vi "button no button.vi"() -> ()   [LabVIEW 2021]
uses:
  <vilib>/myRIO/Instrument Drivers/Onboard IO/PWM/typedefs/PWM Reference.ctl
  <vilib>/myRIO/Common/Instrument Driver Framework/Utilities/typedefs/myRIO Generic Hardware Reference.ctl
  <vilib>/myRIO/Common/Instrument Driver Framework/Utilities/typedefs/Hardware Version Enum.ctl
  <vilib>/myRIO/Common/Instrument Driver Framework/Utilities/typedefs/myRIO v1.0 Reference.ctl
  <vilib>/myRIO/Common/Instrument Driver Framework/Utilities/typedefs/Generic FPGA Reference.ctl
  <vilib>/myRIO/Common/Instrument Driver Framework/myRIO v1.0/PWM/typedefs/PWM Channels Enum.ctl
  <vilib>/myRIO/Instrument Drivers/Onboard IO/PWM/typedefs/PWM Configuration.ctl
  <vilib>/userDefined/High Color/nirio_resource_hc.ctl
  <vilib>/myRIO/Instrument Drivers/Onboard IO/DIO/typedefs/DIO Reference.ctl
  <vilib>/myRIO/Common/Instrument Driver Framework/myRIO v1.0/DIO/typedefs/DIO Channels List.ctl
  <vilib>/myRIO/Common/Instrument Driver Framework/myRIO v1.0/DIO/typedefs/DIO Channels Enum.ctl
  <vilib>/myRIO/Common/Instrument Driver Framework/myRIO v1.0/PWM/vis/myRIO v1.1 Open PWM.vi
  <vilib>/myRIO/Common/Instrument Driver Framework/myRIO v1.0/DIO/vis/myRIO v1.1 Open DIO.vi
  <vilib>/myRIO/Common/Instrument Driver Framework/Utilities/vis/Validate Channels.vi
  <vilib>/myRIO/Common/Instrument Driver Framework/myRIO v1.0/PWM/vis/myRIO v1.0 Reserve PWM.vi
  <vilib>/myRIO/Instrument Drivers/Onboard IO/PWM/vis/Set Duty Cycle and Frequency.vi
  <vilib>/myRIO/Common/Instrument Driver Framework/myRIO v1.0/DIO/vis/myRIO v1.0 Reserve DIO.vi
  <vilib>/myRIO/Common/Instrument Driver Framework/myRIO v1.0/PWM/vis/myRIO v1.0 Close PWM.vi
  <vilib>/myRIO/Common/Instrument Driver Framework/myRIO v1.0/DIO/vis/myRIO v1.0 Close DIO.vi
  <vilib>/myRIO/Common/Instrument Driver Framework/myRIO v1.0/PWM/vis/myRIO v1.0 Build MUX Configuration PWM.vi
  <vilib>/myRIO/Common/Instrument Driver Framework/myRIO v1.0/Resource Manager/vis/myRIO v1.0 Reserve Channel List.vi
  <vilib>/myRIO/Common/Instrument Driver Framework/myRIO v1.0/DIO/vis/myRIO v1.0 Build MUX Configuration DIO.vi
  <vilib>/myRIO/Common/Instrument Driver Framework/myRIO v1.0/PWM/vis/myRIO v1.0 Unreserve PWM.vi
  <vilib>/myRIO/Common/Instrument Driver Framework/myRIO v1.0/DIO/vis/myRIO v1.0 Unreserve DIO.vi
  <vilib>/myRIO/Common/Instrument Driver Framework/myRIO v1.0/Resource Manager/vis/myRIO v1.0 Create Configuration List.vi
  <vilib>/myRIO/Common/Instrument Driver Framework/myRIO v1.0/Resource Manager/vis/myRIO v1.0 Reserve Channel.vi
  <vilib>/myRIO/Common/Instrument Driver Framework/myRIO v1.0/Resource Manager/vis/myRIO v1.0 Unreserve Channel.vi
  <vilib>/myRIO/Common/Instrument Driver Framework/myRIO v1.0/Resource Manager/vis/myRIO v1.0 Unreserve Channel List.vi
  <vilib>/myRIO/Common/Instrument Driver Framework/myRIO v1.0/Resource Manager/vis/myRIO v1.0 Build Mutex Name.vi
  <vilib>/Utility/VariantDataType/GetNumericInfo.vi
  <vilib>/Utility/error.llb/Error Cluster From Error Code.vi
  <vilib>/myRIO/Common/Instrument Driver Framework/myRIO v1.0/myRIO v1.1 Open.vi
  <vilib>/myRIO/Common/Instrument Driver Framework/Utilities/vis/IO Manager.vi
  <vilib>/myRIO/Common/Instrument Driver Framework/Utilities/vis/Configuration Manager.vi
  <vilib>/myRIO/Common/Instrument Driver Framework/myRIO v1.0/Resource Manager/vis/myRIO v1.0 Configure IO.vi
  <vilib>/myRIO/Common/Instrument Driver Framework/myRIO v1.0/myRIO v1.0 Close.vi
  <vilib>/myRIO/Common/Instrument Driver Framework/myRIO v1.0/PWM/vis/myRIO v1.0 Write PWM.vi
  <vilib>/myRIO/Common/Instrument Driver Framework/myRIO v1.0/DIO/vis/myRIO v1.0 Read DIO.vi
  <vilib>/myRIO/Common/Instrument Driver Framework/myRIO v1.0/PWM/vis/myRIO v1.0 Shutdown PWM.vi
  <vilib>/myRIO/Common/Instrument Driver Framework/myRIO v1.0/DIO/vis/myRIO v1.0 Shutdown DIO.vi
  <vilib>/myRIO/Instrument Drivers/Onboard IO/DIO/vis/myRIO DIO Open.xnode
  <vilib>/myRIO/Instrument Drivers/Onboard IO/PWM/vis/myRIO PWM Open.xnode
  <vilib>/myRIO/Instrument Drivers/Onboard IO/DIO/DIO.lvlib
  <vilib>/myRIO/Instrument Drivers/Onboard IO/PWM/PWM.lvlib
panel:
  in  "error in (no error)":errorcluster
  out "and result":bool
  out "x .and. y?":bool
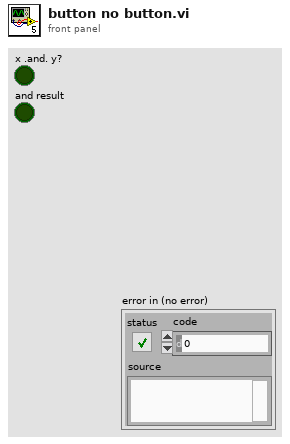
[diagram p1: front panel]
types:
  T1 = typedef "PWM.lvlib/PWM Reference.ctl" = cluster{"myRIO Reference":T2, "PWM Channels Enum":T6, "PWM Configuration":T7}
  T2 = typedef "myRIO Generic Hardware Reference.ctl" = cluster{"myRIO Model":T3, "myRIO Hardware Reference":T4}
  T3 = typedef "Hardware Version Enum.ctl" = enum16{"Unknown", "myRIO-1900", "myRIO-1950", "roboRIO", "NI ELVIS RIO CM", "ELVIS III"}
  T4 = typedef "myRIO v1.0 Reference.ctl" = cluster{"Generic FPGA Reference":T5, "Allow multiple opens":bool}
  T5 = typedef "Generic FPGA Reference.ctl" = refnum<k20>
  T6 = typedef "PWM Channels Enum.ctl" = enum16{"Not Connected", "C/PWM0", "C/PWM1", "A/PWM0", "A/PWM1", "A/PWM2", "A/PWM3", "A/PWM4", "A/PWM5", "A/PWM6", "A/PWM7", "A/PWM8", "A/PWM9", "A/PWM10", "A/PWM11", "A/PWM12", "A/PWM13", "A/PWM14", "A/PWM15", "A/PWM16", "A/PWM17", "A/PWM18", "A/PWM19", "B/PWM0", "B/PWM1", "B/PWM2", "B/PWM3", "B/PWM4", "B/PWM5", "B/PWM6", "B/PWM7", "B/PWM8", "B/PWM9", "B/PWM10", "B/PWM11", "B/PWM12", "B/PWM13", "B/PWM14", "B/PWM15", "B/PWM16", "B/PWM17", "B/PWM18", "B/PWM19", "PWM/PWM0", "PWM/PWM1", "PWM/PWM2", "PWM/PWM3", "PWM/PWM4", "PWM/PWM5", "PWM/PWM6", "PWM/PWM7", "PWM/PWM8", "PWM/PWM9"}
  T7 = typedef "PWM.lvlib/PWM Configuration.ctl" = cluster{"Frequency":dbl, "Duty Cycle":dbl}
  T8 = typedef "DIO.lvlib/DIO Reference.ctl" = cluster{"myRIO Reference":T2, "DIO Channels List":T9}
  T9 = typedef "DIO Channels List.ctl" = T10[]
  T10 = typedef "DIO Channels Enum.ctl" = enum16{"Not Connected", "C/DIO0", "C/DIO1", "C/DIO2", "C/DIO3", "C/DIO4", "C/DIO5", "C/DIO6", "C/DIO7", "A/DIO0", "A/DIO1", "A/DIO2", "A/DIO3", "A/DIO4", "A/DIO5", "A/DIO6", "A/DIO7", "A/DIO8", "A/DIO9", "A/DIO10", "A/DIO11", "A/DIO12", "A/DIO13", "A/DIO14", "A/DIO15", "A/DIO16", "A/DIO17", "A/DIO18", "A/DIO19", "B/DIO0", "B/DIO1", "B/DIO2", "B/DIO3", "B/DIO4", "B/DIO5", "B/DIO6", "B/DIO7", "B/DIO8", "B/DIO9", "B/DIO10", "B/DIO11", "B/DIO12", "B/DIO13", "B/DIO14", "B/DIO15", "B/DIO16", "B/DIO17", "B/DIO18", "B/DIO19", "LED0", "LED1", "LED2", "LED3", "Button0", "DIO/DIO0", "DIO/DIO1", "DIO/DIO2", "DIO/DIO3", "DIO/DIO4", "DIO/DIO5", "DIO/DIO6", "DIO/DIO7", "DIO/DIO8", "DIO/DIO9", "SPI/CS0", "SPI/CS1", "SPI/CS2", "SPI/CS3", "LED RADIO (Green)", "LED RADIO (Red)", "LED COMM (Green)", "LED COMM (Red)", "LED MODE (Green)", "LED MODE (Red)"}
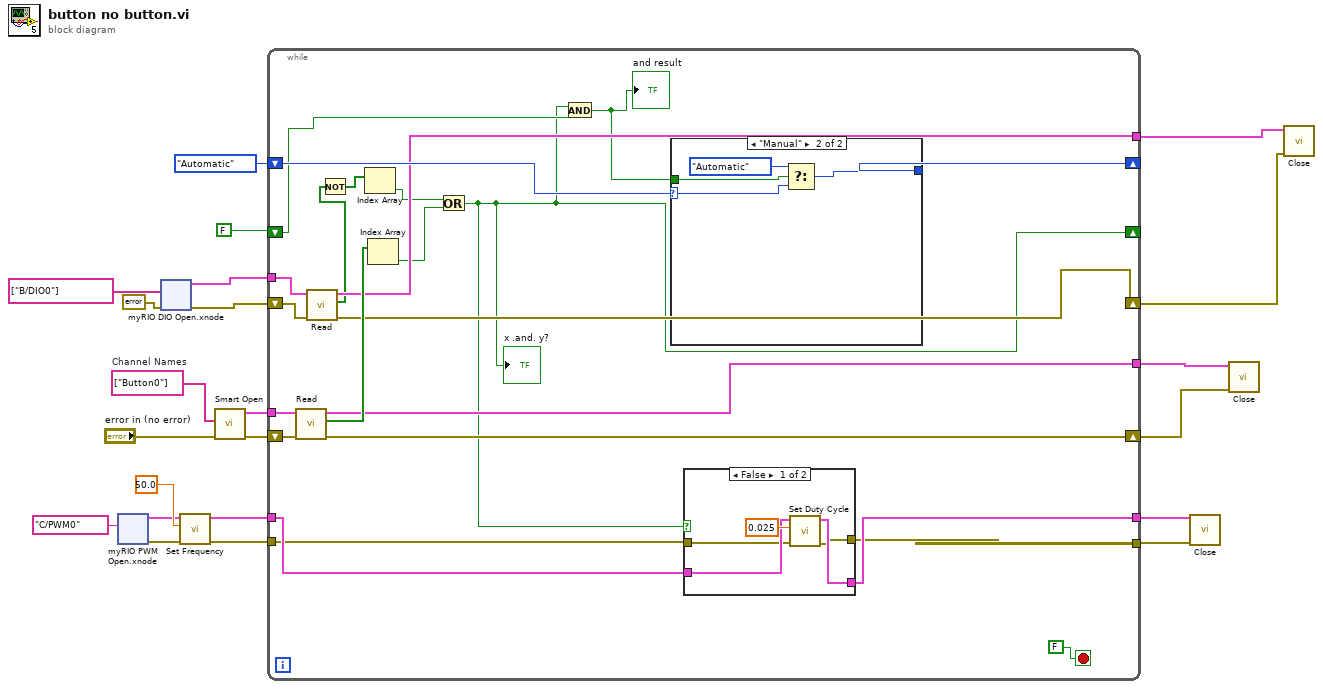
[diagram p0: block diagram]
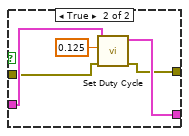
[diagram p2: hidden frame]
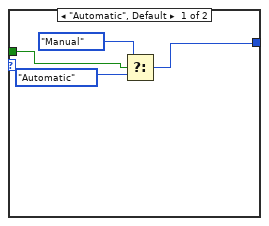
[diagram p3: hidden frame]
diagram:
  w19 = tag[] ["Button0"]  # Channel Names
  n1 = xnode "myRIO PWM Open.xnode"("Channel Name"=tag "C/PWM0") -> ("error out"=w6:errorcluster, "PWM Ref Out"=w7:T1)  [unwired: 2 in]
  n2 = xnode ("myRIO DIO Open.xnode")("error in (no error)"=errorcluster {"status"=FALSE, "code"=0, "source"=""}, "Channel Names"=tag[] ["B/DIO0"]) -> ("error out"=w20:errorcluster, "DIO Ref Out"=w10:T8)  [unwired: 1 in]
  n3 = call <vilib>:"Set Frequency.vi"("error in (no error)"=w6, "Frequency [Hz]"=50.0, "PWM Ref In"=w7) -> ("error out"=w4:errorcluster, "PWM Ref Out"=w5:T1)  [unwired: 6 in]
  n4 = call <vilib>:"Smart Open.vi"("error in (no error)"="error in (no error)", "Channel Names"=w19) -> ("error out"=w22:errorcluster, "DIO Ref Out"=w11:T8)  [unwired: 8 in]
  n5 = while {
    shift-right: [w41] -> w14
    shift-left: w22 -> [w42]
    shift-right: [w34] -> w13
    shift-left: w20 -> [w45]
    tunnel: w10 -> [w44]
    tunnel: w11 -> [w43]
    shift-right: [w38] -> _
    shift-left: enum16{"Automatic", "Manual"}."Automatic" -> [w40]
    tunnel: [w36] -> w16
    tunnel: [w35] -> w15
    tunnel: w5 -> [w24]
    tunnel: w4 -> [w23]
    tunnel: [w26] -> w3
    tunnel: [w25] -> w2
    shift-right: [w27] -> _
    shift-left: FALSE -> [w28]
    stop <- FALSE stop-if-true
    n6 = call <vilib>:"Read.vi"("error in (no error)"=w42, "DIO Ref In"=w43) -> ("error out"=w41:errorcluster, "Values"=w39:bool[], "DIO Ref Out"=w35:T8)  [unwired: 7 in]
    n7 = call <vilib>:"Read.vi"("error in (no error)"=w45, "DIO Ref In"=w44) -> ("error out"=w34:errorcluster, "Values"=w32:bool[], "DIO Ref Out"=w36:T8)  [unwired: 7 in]
    n8 = Not(x=w32) -> (.not. x?=w33:bool[])
    n9 = Index Array "Index Array"(array=w33) -> (element=w29:bool)  [unwired: 1 in]
    n10 = Index Array(array=w39) -> (element=w30:bool)  [unwired: 1 in]
    n11 = Or(x=w29, y=w30) -> (x .or. y?=w27:bool)
    "x .and. y?" <- w27
    n12 = And(x=w27, y=w28) -> (x .and. y?=w31:bool)
    "and result" <- w31
    n13 = case shown="\"Manual\"" w40 {
      selector: w40 -> [_ w61]
      tunnel: [w59 w62] -> w38
      tunnel: w31 -> [w56 w60]
      frame "Automatic", Default {
        n14 = Select(t=enum16{"Automatic", "Manual"}."Manual", s=w56, f=enum16{"Automatic", "Manual"}."Automatic") -> (s? t:f=w59:enum16{"Automatic", "Manual"})
      }
      frame "Manual" {
        n15 = Select(t=enum16{"Automatic", "Manual"}."Automatic", s=w60, f=w61) -> (s? t:f=w62:enum16{"Automatic", "Manual"})
      }
    }
    n16 = case shown="False" w27 {
      tunnel: w24 -> [w49 w54]
      tunnel: w23 -> [w48 w53]
      tunnel: [w47 w52] -> w26
      tunnel: [w46 w51] -> w25
      frame False {
        n17 = call <vilib>:"Set Duty Cycle.vi"("error in (no error)"=w48, "Duty Cycle"=0.025, "PWM Ref In"=w49) -> ("error out"=w46:errorcluster, "PWM Ref Out"=w47:T1)  [unwired: 6 in]
      }
      frame True {
        n18 = call <vilib>:"Set Duty Cycle.vi"("error in (no error)"=w53, "Duty Cycle"=0.125, "PWM Ref In"=w54) -> ("error out"=w51:errorcluster, "PWM Ref Out"=w52:T1)  [unwired: 6 in]
      }
    }
  }
  n19 = call <vilib>:"Close.vi"("error in (no error)"=w2, "PWM Ref In"=w3) -> ()  [unwired: 9 in, 1 out]
  n20 = call <vilib>:"Close.vi"("error in (no error)"=w14, "DIO Ref In"=w15) -> ()  [unwired: 9 in, 1 out]
  n21 = call <vilib>:"Close.vi"("error in (no error)"=w13, "DIO Ref In"=w16) -> ()  [unwired: 9 in, 1 out]
